vi "commSettings.vi"() -> ()   [LabVIEW 2018]
uses:
  TypeDefs/TCPSettings_Global.vi
  TypeDefs/serialSettings_Global.vi
panel:
  in  "Exit":bool
  in  "Save":bool
  in  "Serial Settings":T1={"VISA resource name"="COM1", "baud rate"=9600, "data bits"=8, "parity"=enum."None", "stop bits"=10, "flow control"=0} {"flow control" items=["None"=0, "XON/XOFF"=1, "RTS/CTS"=2, "DTR/DSR"=4]; "stop bits" items=["1.0"=10, "1.5"=15, "2.0"=20]; "data bits" min=5 max=8 step=1; "baud rate" items=["75"=75, "110"=110, "134"=134, "150"=150, "300"=300, "600"=600, "1200"=1200, "1800"=1800, "2400"=2400, "4800"=4800, "7200"=7200, "9600"=9600, "14400"=14400, "19200"=19200, "28800"=28800, "38400"=38400, "56000"=56000, "57600"=57600, "115200"=115200, "128000"=128000, "230400"=230400]}
  in  "TCP Settings":cluster{"service name":string, "port":u16}={"service name"="localhost", "port"=6969}
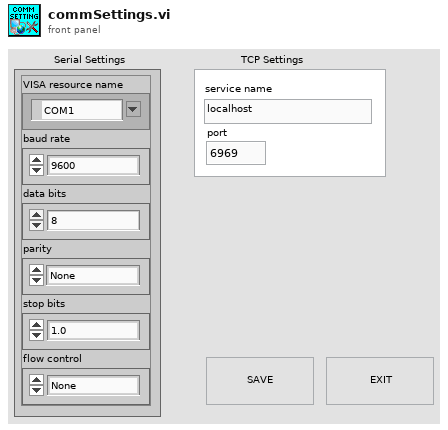
[diagram p1: front panel]
types:
  T1 = cluster{"VISA resource name":refnum<visa-resource-name>, "baud rate":u32, "data bits":u16, "parity":enum16{"None", "Odd", "Even", "Mark", "Space"}, "stop bits":u16, "flow control":u16}
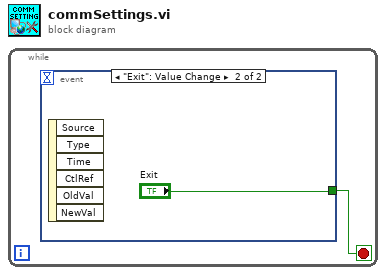
[diagram p0: block diagram]
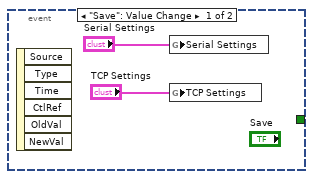
[diagram p2: hidden frame]
diagram:
  n1 = while {
    stop <- w1 stop-if-true
    n2 = event shown="[1] \"Exit\": Value Change" {
      selector: _ -> [_ _]
      dyn-events: _ -> [_ _]
      timeout: _ -> [_ _]
      tunnel: [_ "Exit"] -> w1
      event "Save": Value Change {
        n3 = event-data() -> ()  [unwired: 1 in, 6 out]
        n4 = global write "serialSettings_Global.vi" "Serial Settings"("Serial Settings") -> ()
        n5 = global write "TCPSettings_Global.vi" "TCP Settings"("TCP Settings") -> ()
      }
      event "Exit": Value Change {
        n6 = event-data() -> ()  [unwired: 1 in, 6 out]
      }
    }
  }
